vi "testImportCustomDevice.vi"(8 "error in (no error)":errorcluster, 11 "TestCase in":refnum<class "Routing and Faulting Import Export Unit Tests.lvclass">) -> (0 "error out":errorcluster, 3 "TestCase out":refnum<class "Routing and Faulting Import Export Unit Tests.lvclass">)   [LabVIEW 2017, in "Routing and Faulting Import Export Unit Tests.lvclass"]
uses:
  Routing and Faulting Import Export Unit Tests.lvclass
  Shared/Channel States.ctl
  Shared/Routing State.ctl
  Shared/Connection.ctl
  Routing and Faulting Import Export Unit Tests.lvclass/Routing and Faulting Import Export Unit Tests.ctl
  <userlib>/_OpenG.lib/file/file.llb/Append Path to Root if Relative - Scalar__ogtk.vi
  <vilib>/addons/_JKI Toolkits/VI Tester/TestCase.llb/TestCase.lvclass
  Scripting/Routing and Faulting Scripting.lvlib
  <vilib>/NI/NI VeriStand Custom Device Import and Export Tool/ImportExport.lvlib
  niveristand-custom-device-testing-tools/VeriStandTestUtilities/VeriStandTestUtilities.lvlib
  <vilib>/NI Veristand/Custom Device API/Custom Device API.lvlib
  <vilib>/NI Veristand/Custom Device Tools/Custom Device Utility Library/Custom Device Utility Library.lvlib
  Shared/Routing and Faulting Shared.lvlib
  C:/Program Files (x86)/National Instruments/LabVIEW 2017/vi.lib/addons/_JKI Toolkits/VI Tester/TestCase.llb/TestCase.lvclass
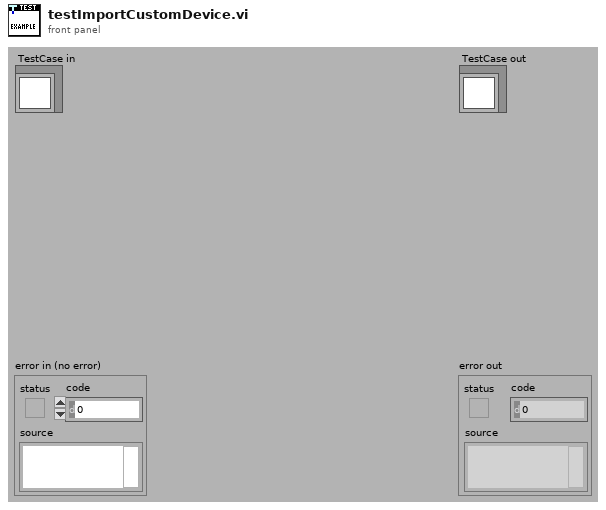
[diagram p1: front panel]
types:
  T1 = typedef "Routing and Faulting Shared.lvlib/Channel States.ctl" = T2[]
  T2 = typedef "Routing and Faulting Shared.lvlib/Routing State.ctl" = cluster{"Name":string, "Description":string, "Value":i32, "Connection List":T3[]}
  T3 = typedef "Routing and Faulting Shared.lvlib/Connection.ctl" = cluster{"Resource":string, "Source":string, "Destination":string}
  T4 = cluster{"Channel Name":string, "Initial State":string, "Description":string, "State Configurations":T1}[]
  T5 = typedef "Custom Device API.lvlib/Custom Device Item Ref.ctl" = u64
  T6 = cluster{"Channel Name":string, "Initial State":string, "Description":string, "State Configurations":T1}
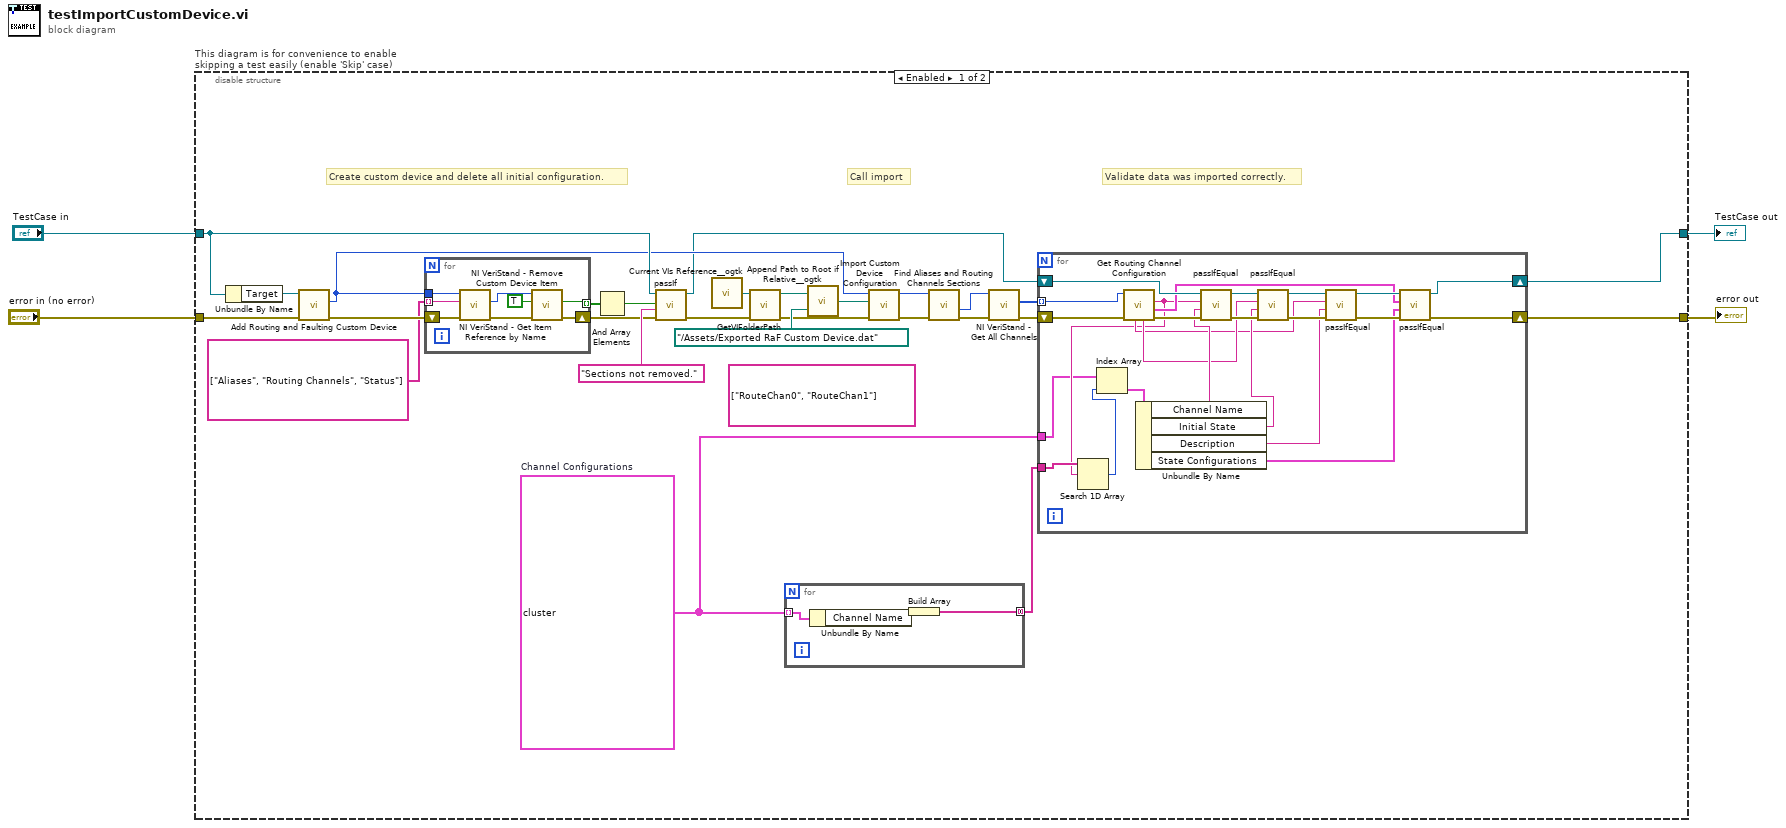
[diagram p0: block diagram]
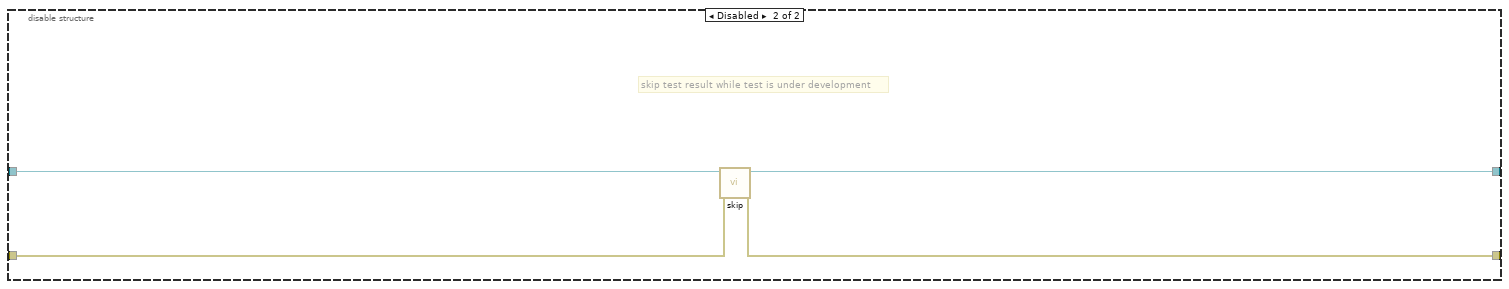
[diagram p2: hidden frame]
diagram:
  n1 = disable-structure "This diagram is for convenience to enable skipping a test easily (enable 'Skip' case)" shown="Enabled" {
    disable-tunnel: "TestCase in" -> [w25 w70]
    disable-tunnel: [w8 w68] -> w1
    disable-tunnel: [w7 w69] -> w3
    disable-tunnel: "error in (no error)" -> [w31 w67]
    frame Enabled {
      w5 = T4 [{"Channel Name"="RouteChan0", "Initial State"="", "Description"="", "State Configurations"=[]}, {"Channel Name"="RouteChan1", "Initial State"="passThrough", "Description"="", "State Configurations"=[{"Name"="addOne", "Description"="addOne description", "Value"=24, "Connection List"=[{"Resource"="2010A", "Source"="J1Ch0p", "Destination"="J2Ch0p"}, {"Resource"="2010B", "Source"="J1Ch0p", "Destination"="J2Ch0p"}]}, {"Name"="passThrough", "Description"="passthrough description", "Value"=23, "Connection List"=[{"Resource"="2010A", "Source"="J1Ch0p", "Destination"="J2Ch16p"}]}]}]  # Channel Configurations
      (unwired) string[] ["RouteChan0", "RouteChan1"]
      # "Validate data was imported correctly."
      # "Call import"
      # "Create custom device and delete all initial configuration."
      n2 = Unbundle By Name(w25) -> ("Target"=w30:refnum<k24>)
      n3 = call "Add Routing and Faulting Custom Device.vi"("error in (no error)"=w31, "Target in"=w30) -> ("error out"=w29:errorcluster, "Routing and Faulting Custom Device Ref"=w16:T5)  [unwired: 7 in, 1 out]
      n4 = for {
        tunnel: w16 -> [w65]
        tunnel: string[] ["Aliases", "Routing Channels", "Status"] -> [w64] mode=indexing
        shift-right: [w60] -> w17
        shift-left: w29 -> [w66]
        tunnel: [w59] -> w28 mode=indexing
        n5 = call <vilib>:"NI VeriStand - Get Item Reference by Name.vi"("error in (no error)"=w66, "Item Name"=w64, "Parent Ref in"=w65) -> ("error out"=w63:errorcluster, "Item Ref"=w62:T5)  [unwired: 5 in, 2 out]
        n6 = call <vilib>:"NI VeriStand - Remove Custom Device Item.vi"("error in (no error)"=w63, "Force Delete (F)"=TRUE, "Item Ref in"=w62) -> ("error out"=w60:errorcluster, "Deleted?"=w59:bool)  [unwired: 7 in]
      }
      n7 = And Array Elements(Boolean array=w28) -> (logical AND=w27:bool)
      n8 = call-dynamic "passIf.vi"("error in (no error)"=w17, "message (\"\")"="Sections not removed." ("message (\"\")"), "pass"=w27, "TestCase in"=w25) -> ("error out"=w20:errorcluster, "TestCase out"=w9:refnum<class "Routing and Faulting Import Export Unit Tests.lvclass">)  [unwired: 6 in]
      n9 = call <userlib>:"Current VIs Reference__ogtk.vi"() -> ("Current VI's reference"=w24:refnum<vi>)  [unwired: 5 in]
      n10 = call "GetVIFolderPath.vi"("error in (no error)"=w20, "VI Reference in"=w24) -> ("error out"=w19:errorcluster, "VI Folder Path out"=w23:path)  [unwired: 8 in]
      n11 = for {
        tunnel: w5 -> [w34] mode=indexing
        tunnel: [w32] -> w6 mode=concatenating
        n12 = Unbundle By Name(w34) -> ("Channel Name"=w33:string)
        n13 = Build Array(w33) -> (w32:string[])
      }
      n14 = call-poly <userlib>:"Append Path to Root if Relative__ogtk.vi"("Absolute or Relative Path"=path "../Assets/Exported RaF Custom Device.dat", "Root Path"=w23) -> ("Absolute or Appended Path"=w21:path)
      n15 = call <vilib>:"Import Custom Device Configuration.vi"("error in (no error)"=w19, "Path"=w21, "NodeID"=w16) -> ("error out"=w15:errorcluster, "NodeID out"=w14:u64)  [unwired: 6 in, 1 out]
      n16 = call "Find Aliases and Routing Channels Sections.vi"("error in (no error)"=w15, "Routing and Faulting Custom Device Ref in"=w14) -> ("error out"=w13:errorcluster, "Routing Channels Ref"=w12:T5)  [unwired: 6 in, 2 out]
      n17 = call <vilib>:"NI VeriStand - Get All Channels.vi"("error in"=w13, "Section Ref in"=w12) -> ("error out"=w11:errorcluster, "Channel Refs"=w10:T5[])  [unwired: 6 in, 2 out]
      n18 = for {
        tunnel: w10 -> [w57] mode=indexing
        shift-right: [w48] -> w8
        shift-left: w9 -> [w55]
        shift-right: [w47] -> w7
        shift-left: w11 -> [w58]
        tunnel: w6 -> [w39]
        tunnel: w5 -> [w37]
        n19 = call "Get Routing Channel Configuration.vi"("error in (no error)"=w58, "Channel Ref in"=w57) -> ("error out"=w56:errorcluster, "State and Connections List"=w41:T1, "Channel Name"=w38:string, "Initial State"=w45:string, "Description"=w43:string)  [unwired: 4 in, 1 out]
        n20 = Search 1D Array(1D array=w39, element=w38) -> (index of element=w36:i32)  [unwired: 1 in]
        n21 = Index Array(array=w37, index=w36) -> (element=w35:T6)
        n22 = Unbundle By Name(w35) -> ("Channel Name"=w46:string, "Initial State"=w44:string, "Description"=w42:string, "State Configurations"=w40:T1)
        n23 = call-dynamic "passIfEqual.vi"("error in (no error)"=w56, "y"=w46, "x"=w38, "TestCase in"=w55) -> ("error out"=w54:errorcluster, "TestCase out"=w51:refnum<class "Routing and Faulting Import Export Unit Tests.lvclass">)  [unwired: 6 in]
        n24 = call-dynamic "passIfEqual.vi"("error in (no error)"=w54, "y"=w44, "x"=w45, "TestCase in"=w51) -> ("error out"=w53:errorcluster, "TestCase out"=w50:refnum<class "Routing and Faulting Import Export Unit Tests.lvclass">)  [unwired: 6 in]
        n25 = call-dynamic "passIfEqual.vi"("error in (no error)"=w53, "y"=w42, "x"=w43, "TestCase in"=w50) -> ("error out"=w52:errorcluster, "TestCase out"=w49:refnum<class "Routing and Faulting Import Export Unit Tests.lvclass">)  [unwired: 6 in]
        n26 = call-dynamic "passIfEqual.vi"("error in (no error)"=w52, "y"=w40, "x"=w41, "TestCase in"=w49) -> ("error out"=w47:errorcluster, "TestCase out"=w48:refnum<class "Routing and Faulting Import Export Unit Tests.lvclass">)  [unwired: 6 in]
      }
    }
    frame Disabled {
      # "skip test result while test is under development"
      n27 = call <vilib>:"skip.vi"("error in (no error)"=w67, "TestCase in"=w70) -> ("error out"=w69:errorcluster, "TestCase out"=w68:refnum<class "Routing and Faulting Import Export Unit Tests.lvclass">)  [unwired: 8 in]
    }
  }
  "error out" <- w3
  "TestCase out" <- w1
